vi "Log Message core.vi"(7 "Time Stamp":timestamp, 8 "error in (no error)":errorcluster, 9 "Message":refnum<class "Message.lvclass">, 10 "Receiving Actor":refnum<class "Message Enqueuer.lvclass">, 11 "Classic Monitor in":refnum<class "Classic Monitor.lvclass">) -> (0 "error out":errorcluster, 3 "Classic Monitor out":refnum<class "Classic Monitor.lvclass">)   [LabVIEW 2023, in "Monitored Actor.lvlib" / "Classic Monitor.lvclass"]
uses:
  Classic Monitor.lvclass
  builds/Engine/Actor Framework.lvlibp/1abvi3w/vi.lib/ActorFramework/Message/Message.lvclass
  builds/Engine/Actor Framework.lvlibp/1abvi3w/vi.lib/ActorFramework/Message Enqueuer/Message Enqueuer.lvclass
  Classic Monitor.lvclass/Classic Monitor.ctl
  Logger/Classic Logger Messages/New Message Msg/New Message Msg.lvclass
  Monitored Actor/Monitored Actor Messages/Disable Message Logging Msg/Disable Message Logging Msg.lvclass
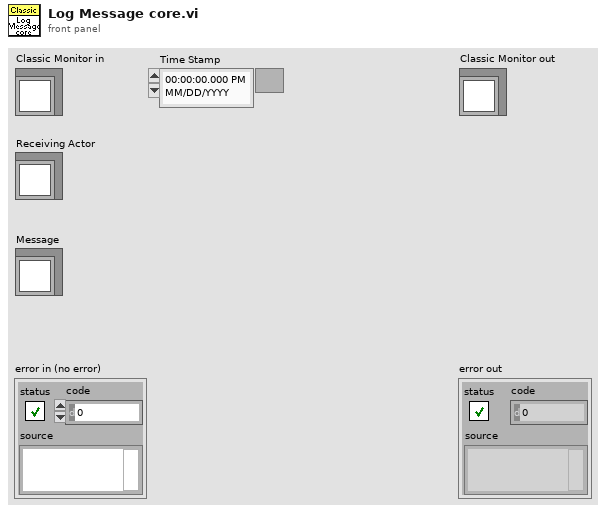
[diagram p1: front panel]
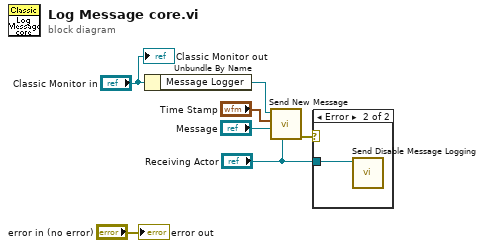
[diagram p0: block diagram]
diagram:
  n1 = Unbundle By Name("Classic Monitor in") -> ("Message Logger"=w5:refnum<class "Message Enqueuer.lvclass">)
  n2 = call "Send New Message.vi"("Receiving Actor"="Receiving Actor", "Message"="Message", "Time Stamp"="Time Stamp", "Message Enqueuer in"=w5) -> ("error out"=w2:errorcluster)  [unwired: 6 in, 1 out]
  n3 = case shown="Error" w2 {
    tunnel: "Receiving Actor" -> [_ w8]
    frame No Error {
    }
    frame Error {
      n4 = call "Send Disable Message Logging.vi"("Message Enqueuer in"=w8) -> ()  [unwired: 9 in, 2 out]
    }
  }
  "error out" <- "error in (no error)"
  "Classic Monitor out" <- "Classic Monitor in"
